vi "BRig_Host_dataRunState__dataTS_findRow.vi"(8 "input_nTrial":u16, 10 "input_idx":i32[](array[numeric]), 11 "input_dataTS":u16[][](array[numeric])) -> (2 "output_row_dataTS":i32, 3 "output_I_row_dataTS":bool)   [LabVIEW 2014]
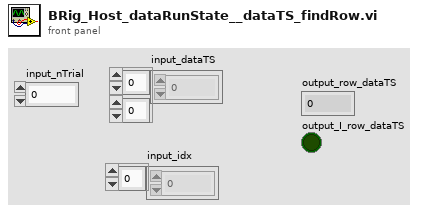
[diagram p1: front panel]
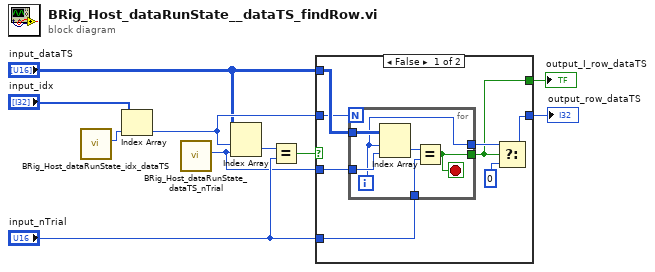
[diagram p0: block diagram]
diagram:
  n1 = call "BRig_Host_dataRunState_idx_dataTS.vi"() -> ("output_idx_dataTS"=w10:i32)  [unwired: 11 in]
  n2 = Index Array(array="input_idx", index=w10) -> (element=w6:i32)
  n3 = call "BRig_Host_dataRunState_dataTS_nTrial.vi"() -> ("output_idx_dataTS_nTrial"=w2:i32)  [unwired: 11 in]
  n4 = Index Array(array="input_dataTS", index (row)=w6, index (col)=w2) -> (element=w8:u16)
  n5 = Equal?(x=w8, y="input_nTrial") -> (x = y?=w7:bool)
  n6 = case shown="False" w7 {
    selector: w7 -> [_ w25]
    tunnel: w6 -> [w15 w26]
    tunnel: [w13 w26] -> w5
    tunnel: "input_nTrial" -> [w16 _]
    tunnel: "input_dataTS" -> [w17 _]
    tunnel: w2 -> [w18 _]
    tunnel: [w11 w25] -> w1
    frame False {
      n7 = for {
        N: w15 -> [_]
        tunnel: w18 -> [w23]
        tunnel: w17 -> [w22]
        tunnel: w16 -> [w21]
        tunnel: [w20] -> w11
        tunnel: [w19] -> w14
        i -> [w19]
        stop <- w20 stop-if-true
        n8 = Index Array(array=w22, index (row)=w19, index (col)=w23) -> (element=w24:u16)
        n9 = Equal?(x=w24, y=w21) -> (x = y?=w20:bool)
      }
      n10 = Select(t=w14, s=w11, f=0) -> (s? t:f=w13:i32)
    }
    frame True {
    }
  }
  "output_row_dataTS" <- w5
  "output_I_row_dataTS" <- w1
